vi "Buck Converter Efficiency Test.vi"(6 "DMM Session":refnum<k15>="Dev1", 8 "error in (no error)":errorcluster, 9 "Channel List":string[](array[string]), 10 "DCPower Session":refnum<k15>[](array[refnum]), 11 "measurement configuration":T3={"Vin Pin Name"="", "Source Voltage Level (V)"=3.0, "Source Current Limit (A)"=1.0, "Eload Pin Name"="", "Load Voltage Limit (V)"=5.0, "Points"=10, "Current Load Level Start"=0.1, "Current Load Level Stop"=1.0, "Vout Pin Name"="", "Range"=10.0, "Resolution in Digits"=enum."5 1/2"} {"Range" min=0.0 step=0.1; "Current Load Level Stop" min=1.0; "Points" min=1; "Source Current Limit (A)" format="%#_6p"; "Source Voltage Level (V)" format="%#_6p"}) -> (0 "error out":errorcluster, 3 "measurement results":T1)   [LabVIEW 2024, in "PMIC_Efficiency_DMM.lvlib"]
uses:
  PMIC_Efficiency_DMM.lvlib
  Measurement Configuration.ctl
  measurementlink-labview-examples-2.0.0.1/NI-DMM Measurement/NIDmmMeasurement/ResolutionInDigits.ctl
  Measurement Results.ctl
  <vilib>/gRPC/Generated APIs/ni/protobuf/types/RPC Messages/ni_protobuf_types_DoubleXYData.ctl
  <instrlib>/niDMM/nidmm.llb/niDMM Resolution in Digits.ctl
  <instrlib>/niDCPower/nidcpower.llb/niDCPower Output Function.ctl
  <instrlib>/niDCPower/nidcpower.llb/niDCPower Source Mode.ctl
  <instrlib>/niDCPower/nidcpower.llb/niDCPower Measurement Type.ctl
  <instrlib>/niDMM/nidmm.llb/niDMM Function.ctl
  <instrlib>/niDMM/nidmm.llb/niDMM Configure Measurement Digits.vi
  <vilib>/gRPC/Generated APIs/ni/protobuf/types/ni.protobuf.types.lvlib
  measurementlink-labview-examples-2.0.0.1/NI-DMM Measurement/NIDmmMeasurement/NIDmmMeasurement.lvlib
panel:
  out "Over Range?":bool
  out "Iin":dbl[](graph)
  out "Vin":dbl[](graph)
  out "Iout":dbl[](graph)
  out "Vout":dbl[](graph)
  out "Efficiency":cluster{dbl[], dbl[]}(graph)
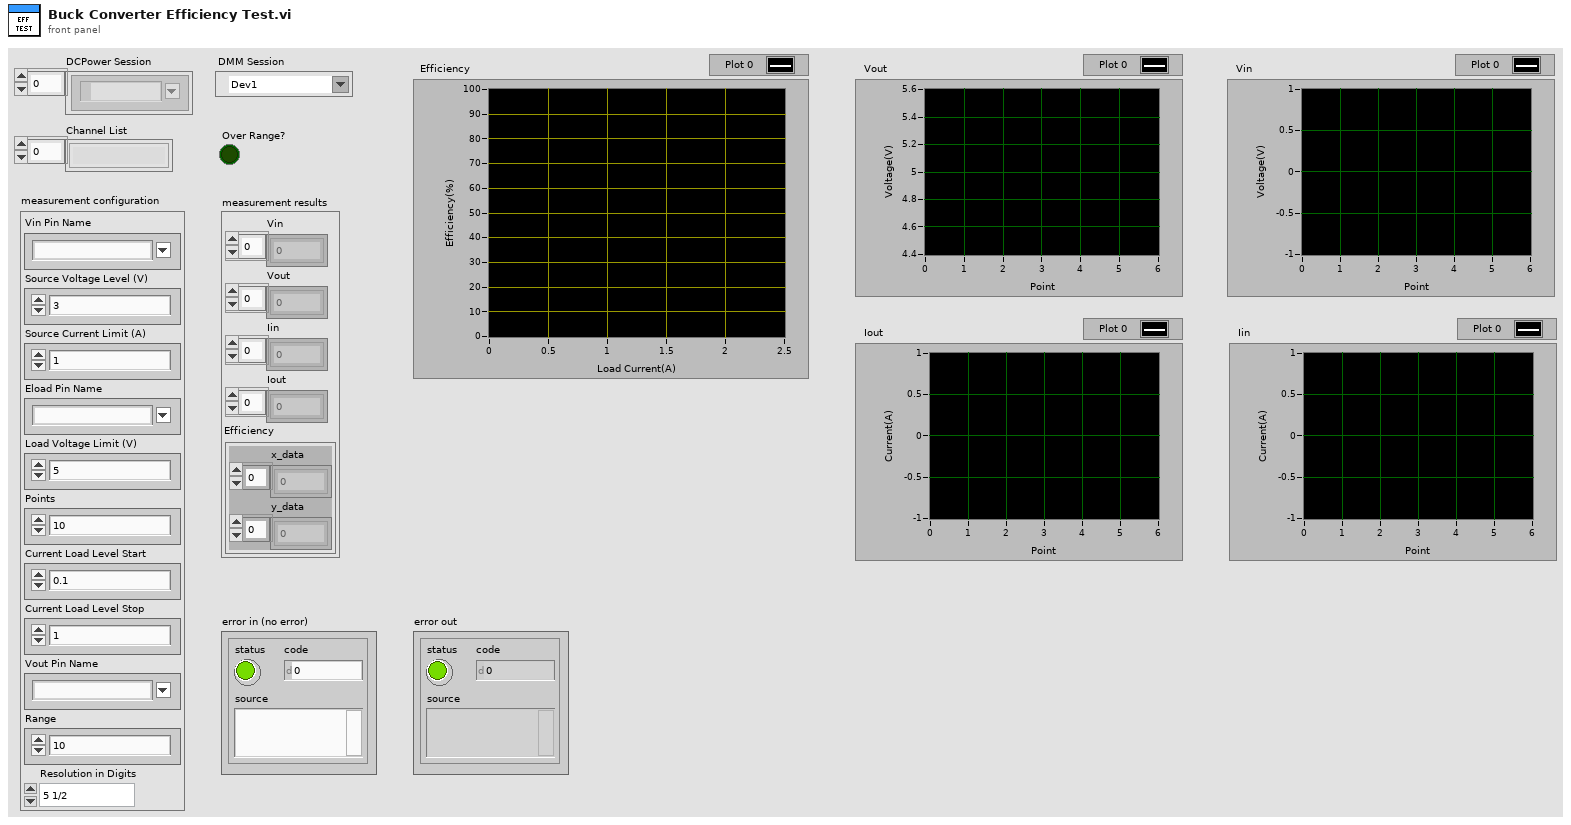
[diagram p1: front panel]
types:
  T1 = typedef "PMIC_Efficiency_DMM.lvlib/Measurement Results.ctl" = cluster{"Vin":dbl[], "Vout":dbl[], "Iin":dbl[], "Iout":dbl[], "Efficiency":T2}
  T2 = typedef "ni.protobuf.types.lvlib/ni_protobuf_types_DoubleXYData.ctl" = cluster{"x_data":dbl[], "y_data":dbl[]}
  T3 = typedef "PMIC_Efficiency_DMM.lvlib/Measurement Configuration.ctl" = cluster{"Vin Pin Name":string, "Source Voltage Level (V)":dbl, "Source Current Limit (A)":dbl, "Eload Pin Name":string, "Load Voltage Limit (V)":dbl, "Points":i32, "Current Load Level Start":dbl, "Current Load Level Stop":dbl, "Vout Pin Name":string, "Range":dbl, "Resolution in Digits":T4}
  T4 = typedef "NIDmmMeasurement.lvlib/ResolutionInDigits.ctl" = enum32{"3 1/2", "4 1/2", "5 1/2", "6 1/2", "7 1/2"}
  T5 = typedef "niDMM Function.ctl" = enum16{"DC Volts", "AC Volts", "DC Current", "AC Current", "2-wire Resistance", "4-wire Resistance", "Diode", "Frequency", "Period", "AC Volts DC Coupled", "Capacitance", "Inductance", "Temperature"}
  T6 = typedef "niDMM Resolution in Digits.ctl" = dbl
  T7 = typedef "niDCPower Measurement Type.ctl" = i32
  T8 = typedef "niDCPower Source Mode.ctl" = i32
  T9 = typedef "niDCPower Output Function.ctl" = i32
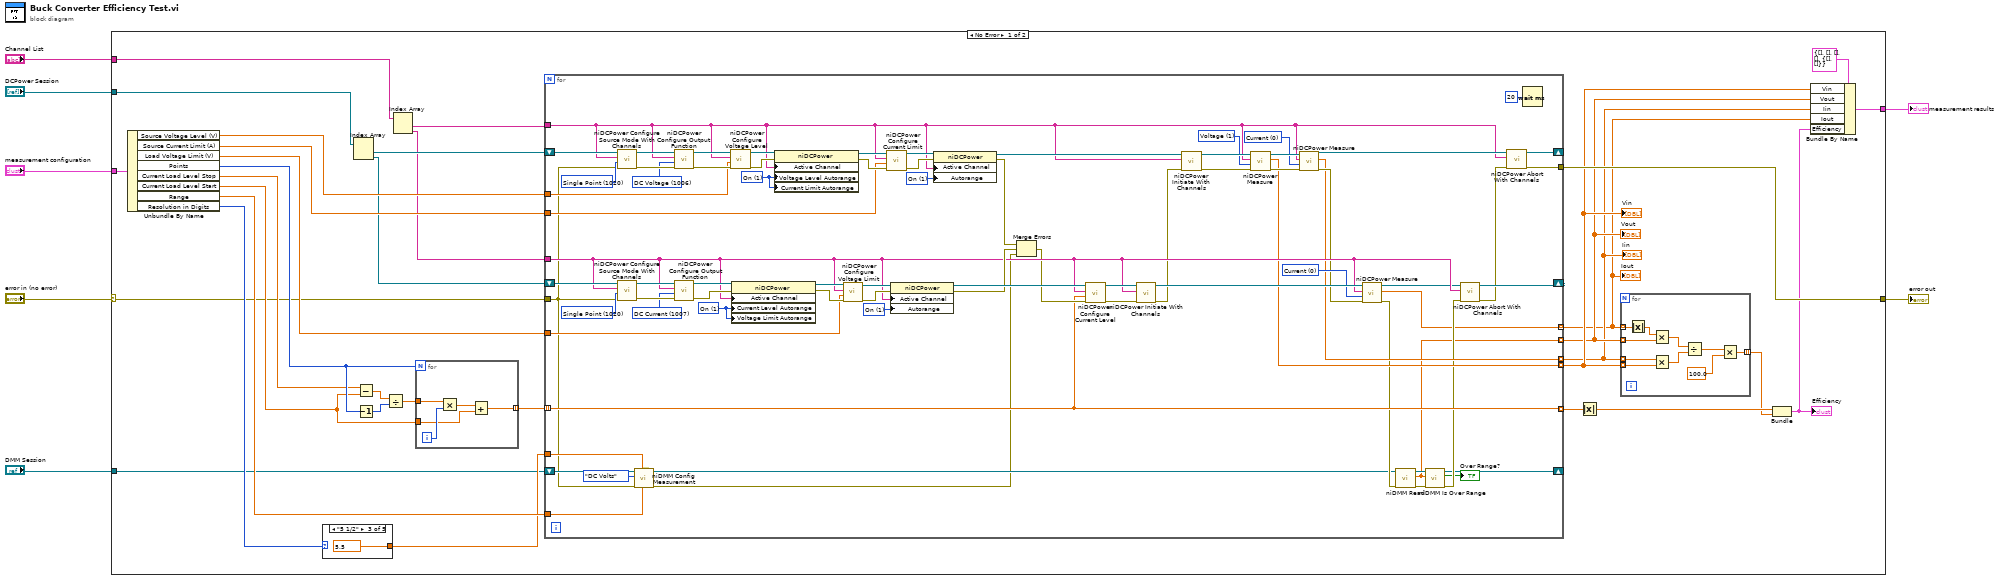
[diagram p0: block diagram]
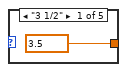
[diagram p2: hidden frame]
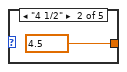
[diagram p3: hidden frame]
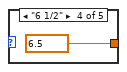
[diagram p4: hidden frame]
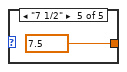
[diagram p5: hidden frame]
diagram:
  n1 = case shown="No Error" "error in (no error)" {
    selector: "error in (no error)" -> [w24 w136]
    tunnel: "measurement configuration" -> [w34 _]
    tunnel: [w23 w136] -> w5
    tunnel: "DCPower Session" -> [w20 _]
    tunnel: "DMM Session" -> [w19 _]
    tunnel: [w18 _] -> w2
    tunnel: "Channel List" -> [w11 _]
    frame No Error {
      n2 = Unbundle By Name(w34) -> ("Source Voltage Level (V)"=w33:dbl, "Source Current Limit (A)"=w32:dbl, "Load Voltage Limit (V)"=w31:dbl, "Points"=w30:i32, "Current Load Level Stop"=w29:dbl, "Current Load Level Start"=w28:dbl, "Range"=w26:dbl, "Resolution in Digits"=w27:T4)
      n3 = case shown="\"5 1/2\"" w27 {
        tunnel: [w41 w42 w43 w44 w45] -> w25
        frame "3 1/2" {
          w41 = T6 3.5 items=["3 1/2"=3.5, "4 1/2"=4.5, "5 1/2"=5.5, "6 1/2"=6.5, "7 1/2"=7.5] ("Resolution in Digits")
        }
        frame "4 1/2" {
          w42 = T6 4.5 items=["3 1/2"=3.5, "4 1/2"=4.5, "5 1/2"=5.5, "6 1/2"=6.5, "7 1/2"=7.5] ("Resolution in Digits")
        }
        frame "5 1/2" {
          w43 = T6 5.5 items=["3 1/2"=3.5, "4 1/2"=4.5, "5 1/2"=5.5, "6 1/2"=6.5, "7 1/2"=7.5] ("Resolution in Digits")
        }
        frame "6 1/2" {
          w44 = T6 6.5 items=["3 1/2"=3.5, "4 1/2"=4.5, "5 1/2"=5.5, "6 1/2"=6.5, "7 1/2"=7.5] ("Resolution in Digits")
        }
        frame "7 1/2" {
          w45 = T6 7.5 items=["3 1/2"=3.5, "4 1/2"=4.5, "5 1/2"=5.5, "6 1/2"=6.5, "7 1/2"=7.5] ("Resolution in Digits")
        }
      }
      n4 = Index Array(array=w20) -> (element #1=w22:refnum<k15>, element #2=w21:refnum<k15>)  [unwired: 2 in]
      n5 = Subtract(x=w29, y=w28) -> (x-y=w40:dbl)
      n6 = Decrement(x=w30) -> (x-1=w39:i32)
      n7 = Divide(x=w40, y=w39) -> (x/y=w38:dbl)
      n8 = Index Array(array=w11) -> (element #1=w10:string, element #2=w9:string)  [unwired: 2 in]
      n9 = for {
        N: w30 -> [_]
        tunnel: w38 -> [w135]
        tunnel: w28 -> [w132]
        tunnel: [w131] -> w37 mode=indexing
        i -> [w134]
        n10 = Multiply(x=w135, y=w134) -> (x*y=w133:dbl)
        n11 = Add(x=w133, y=w132) -> (x+y=w131:dbl)
      }
      n12 = for {
        shift-right: [w92] -> _
        shift-left: w22 -> [w130]
        shift-right: [w91] -> _
        shift-left: w21 -> [w113]
        tunnel: [w62] -> w16 mode=indexing
        tunnel: [w89] -> w23
        tunnel: w32 -> [w86]
        tunnel: w33 -> [w85]
        tunnel: w10 -> [w84]
        tunnel: w9 -> [w79]
        tunnel: w31 -> [w83]
        tunnel: [w75] -> w17 mode=indexing
        tunnel: [w74] -> w15 mode=indexing
        tunnel: w37 -> [w73] mode=indexing
        tunnel: [w73] -> w36 mode=indexing
        shift-right: [w64] -> _
        shift-left: w19 -> [w71]
        tunnel: w26 -> [w63]
        tunnel: [w61] -> w14 mode=indexing
        tunnel: w25 -> [w59]
        tunnel: w24 -> [w58]
        w94 = T7 0 items=["Current", "Voltage"] ("measurement type")
        w96 = T7 0 items=["Current", "Voltage"] ("measurement type")
        w97 = T7 1 items=["Current", "Voltage"] ("measurement type")
        w107 = 1 items=["Off", "On"] ("Measurement:Autorange")
        w108 = 1 items=["Off", "On"] ("Source:DC Voltage:Voltage Level Autorange")
        w109 = T8 1020 items=["Single Point"=1020, "Sequence"=1021] ("source mode")
        w110 = T9 1007 items=["DC Voltage"=1006, "DC Current"=1007, "Pulse Voltage"=1049, "Pulse Current"=1050] ("output function")
        w115 = 1 items=["Off", "On"] ("Measurement:Autorange")
        w119 = 1 items=["Off", "On"] ("Source:DC Voltage:Voltage Level Autorange")
        w122 = T8 1020 items=["Single Point"=1020, "Sequence"=1021] ("source mode")
        w123 = T9 1006 items=["DC Voltage"=1006, "DC Current"=1007, "Pulse Voltage"=1049, "Pulse Current"=1050] ("output function")
        # "3"
        # "2"
        n13 = call <instrlib>:"niDCPower Configure Source Mode With Channels.vi"("error in (no error)"=w58, "source mode"=w122, "channel name"=w84, "instrument handle"=w130) -> ("error out"=w128:errorcluster, "instrument handle out"=w129:refnum<k15>)  [unwired: 6 in]
        n14 = call <instrlib>:"niDCPower Configure Source Mode With Channels.vi"("error in (no error)"=w58, "source mode"=w109, "channel name"=w79, "instrument handle"=w113) -> ("error out"=w111:errorcluster, "instrument handle out"=w112:refnum<k15>)  [unwired: 6 in]
        n15 = call-poly <instrlib>:"niDMM Config Measurement.vi"("Range"=w63, "Resolution in Digits"=w59, "error in (no error)"=w58, "Function"=niDMM_Function."DC Volts", "instrument handle"=w71) -> ("error out"=w65:errorcluster, "instrument handle out"=w66:refnum<k15>)  [unwired: 5 in]
        n16 = call <instrlib>:"niDCPower Configure Output Function.vi"("error in (no error)"=w128, "output function"=w123, "channel name"=w84, "instrument handle"=w129) -> ("error out"=w126:errorcluster, "instrument handle out"=w127:refnum<k15>)  [unwired: 6 in]
        n17 = call <instrlib>:"niDCPower Configure Output Function.vi"("error in (no error)"=w111, "output function"=w110, "channel name"=w79, "instrument handle"=w112) -> ("error out"=w101:errorcluster, "instrument handle out"=w102:refnum<k15>)  [unwired: 6 in]
        n18 = call <instrlib>:"niDCPower Configure Voltage Level.vi"("error in (no error)"=w126, "voltage level"=w85, "channel name"=w84, "instrument handle"=w127) -> ("error out"=w124:errorcluster, "instrument handle out"=w125:refnum<k15>)  [unwired: 6 in]
        n19 = property class="niDCPower"(reference=w102, error in=w101, "Active Channel"=w79, "Current Level Autorange"=w108, "Voltage Limit Autorange"=w108) -> (reference out=w106:refnum<k15>, error out=w104:errorcluster)
        n20 = property class="niDCPower"(reference=w125, error in=w124, "Active Channel"=w84, "Voltage Level Autorange"=w119, "Current Limit Autorange"=w119) -> (reference out=w121:refnum<k15>, error out=w120:errorcluster)
        n21 = call <instrlib>:"niDCPower Configure Voltage Limit.vi"("error in (no error)"=w104, "voltage limit"=w83, "channel name"=w79, "instrument handle"=w106) -> ("error out"=w103:errorcluster, "instrument handle out"=w105:refnum<k15>)  [unwired: 6 in]
        n22 = call <instrlib>:"niDCPower Configure Current Limit.vi"("error in (no error)"=w120, "current limit"=w86, "channel name"=w84, "instrument handle"=w121) -> ("error out"=w116:errorcluster, "instrument handle out"=w118:refnum<k15>)  [unwired: 6 in]
        n23 = property class="niDCPower"(reference=w105, error in=w103, "Active Channel"=w79, "Autorange"=w107) -> (reference out=w82:refnum<k15>, error out=w80:errorcluster)
        n24 = property class="niDCPower"(reference=w118, error in=w116, "Active Channel"=w84, "Autorange"=w115) -> (reference out=w117:refnum<k15>, error out=w81:errorcluster)
        n25 = Merge Errors(w81, w80, w65) -> (w78:errorcluster)
        n26 = call <instrlib>:"niDCPower Configure Current Level.vi"("error in (no error)"=w78, "current level"=w73, "channel name"=w79, "instrument handle"=w82) -> ("error out"=w99:errorcluster, "instrument handle out"=w100:refnum<k15>)  [unwired: 6 in]
        n27 = call <instrlib>:"niDCPower Initiate With Channels.vi"("error in (no error)"=w99, "channel name"=w79, "instrument handle"=w100) -> ("error out"=w77:errorcluster, "instrument handle out"=w95:refnum<k15>)  [unwired: 7 in]
        n28 = call <instrlib>:"niDCPower Initiate With Channels.vi"("error in (no error)"=w77, "channel name"=w84, "instrument handle"=w117) -> ("error out"=w90:errorcluster, "instrument handle out"=w114:refnum<k15>)  [unwired: 7 in]
        n29 = call <instrlib>:"niDCPower Measure.vi"("error in (no error)"=w90, "measurement type"=w97, "channel name"=w84, "instrument handle"=w114) -> ("error out"=w93:errorcluster, "measurement"=w75:dbl, "instrument handle out"=w98:refnum<k15>)  [unwired: 5 in]
        n30 = call <instrlib>:"niDCPower Measure.vi"("error in (no error)"=w93, "measurement type"=w96, "channel name"=w84, "instrument handle"=w98) -> ("error out"=w76:errorcluster, "measurement"=w74:dbl, "instrument handle out"=w87:refnum<k15>)  [unwired: 5 in]
        n31 = call <instrlib>:"niDCPower Measure.vi"("error in (no error)"=w76, "measurement type"=w94, "channel name"=w79, "instrument handle"=w95) -> ("error out"=w68:errorcluster, "measurement"=w61:dbl, "instrument handle out"=w60:refnum<k15>)  [unwired: 5 in]
        n32 = call <instrlib>:"niDMM Read.vi"("error in (no error)"=w68, "instrument handle"=w66) -> ("error out"=w69:errorcluster, "Measurement"=w62:dbl, "instrument handle out"=w70:refnum<k15>)  [unwired: 7 in]
        n33 = call <instrlib>:"niDMM Is Over Range.vi"("error in (no error)"=w69, "Measurement"=w62, "instrument handle"=w70) -> ("error out"=w67:errorcluster, "Over Range?"=→"Over Range?":bool, "instrument handle out"=w64:refnum<k15>)  [unwired: 6 in]
        n34 = call <instrlib>:"niDCPower Abort With Channels.vi"("error in (no error)"=w67, "channel name"=w79, "instrument handle"=w60) -> ("error out"=w88:errorcluster, "instrument handle out"=w91:refnum<k15>)  [unwired: 7 in]
        n35 = call <instrlib>:"niDCPower Abort With Channels.vi"("error in (no error)"=w88, "channel name"=w84, "instrument handle"=w87) -> ("error out"=w89:errorcluster, "instrument handle out"=w92:refnum<k15>)  [unwired: 7 in]
        n36 = Wait (ms)(milliseconds to wait=u32 20) -> ()  [unwired: 1 out]
      }
      "Vout" <- w16
      "Iout" <- w14
      "Vin" <- w17
      "Iin" <- w15
      n37 = Absolute Value(x=w36) -> (abs(x)=w35:dbl[])
      n38 = for {
        tunnel: w16 -> [w55] mode=indexing
        tunnel: [w49] -> w8 mode=indexing
        tunnel: w15 -> [w48] mode=indexing
        tunnel: w17 -> [w47] mode=indexing
        tunnel: w14 -> [w46] mode=indexing
        n39 = Absolute Value(x=w46) -> (abs(x)=w52:dbl)
        n40 = Multiply(x=w52, y=w55) -> (x*y=w54:dbl)
        n41 = Multiply(x=w48, y=w47) -> (x*y=w53:dbl)
        n42 = Divide(x=w54, y=w53) -> (x/y=w51:dbl)
        n43 = Multiply(x=w51, y=100.0) -> (x*y=w49:dbl)
      }
      n44 = Bundle(w35, w8) -> (w12:cluster{dbl[], dbl[]})  [unwired: 1 in]
      "Efficiency" <- w12
      n45 = Bundle By Name(cluster=T1 {"Vin"=[], "Vout"=[], "Iin"=[], "Iout"=[], "Efficiency"={"x_data"=[], "y_data"=[]}} ("measurement results"), "Vin"=w17, "Vout"=w16, "Iin"=w15, "Iout"=w14, "Efficiency"=w12) -> (w18:T1)
    }
    frame Error {
    }
  }
  "error out" <- w5
  "measurement results" <- w2
